vi "TestSSM.vi"(7 "TestBase.lvclass":refnum<class "TestBase.lvclass">, 10 "Script":string[](array[string])=["SamplerInitialize", "SamplerFetch,5000", "SyncSetTimedTrigger,Timed_1,0.1,0.1", "SamplerGetSamples", "Stop"], 11 "ModuleIDs":i32[](array[numeric])=[4140002, 4140002, 4140002, 4140002]) -> (0 "ErrorArray":errorcluster[](array[cluster]), 3 "Data":variant=variant(cluster{"dReadingArray":dbl[], "iActualPts":i32, "Timestamp":dbl}[] [{"dReadingArray"=array[9600 elements], "iActualPts"=9600, "Timestamp"=3606475867.981776}, {"dReadingArray"=array[9600 elements], "iActualPts"=9600, "Timestamp"=3606475867.981776}, {"dReadingArray"=array[9600 elements], "iActualPts"=9600, "Timestamp"=3606475867.981776}, {"dReadingArray"=array[9600 elements], "iActualPts"=9600, "Timestamp"=3606475867.981776}, {"dReadingArray"=array[9600 elements], "iActualPts"=9600, "Timestamp"=3606475867.981776}, {"dReadingArray"=array[9600 elements], "iActualPts"=9600, "Timestamp"=3606475867.981776}]))   [LabVIEW 2014, in "TestBase.lvclass"]
uses:
  TestBase.lvclass
  TestBase.lvclass/TestBase.ctl
  Accessors/Write ModuleIDs.vi
  Accessors/Write PluginPathArray.vi
  LV_Ini/Ini_lib.lvlib
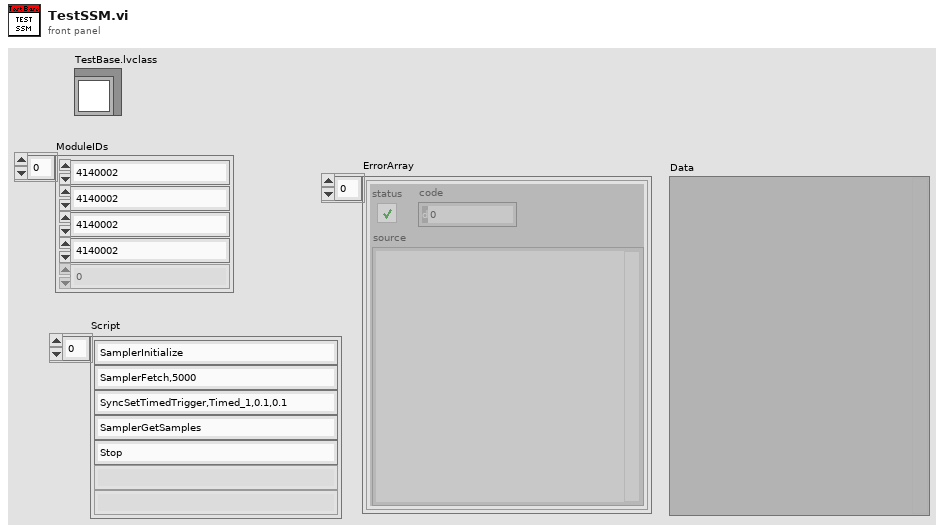
[diagram p1: front panel]
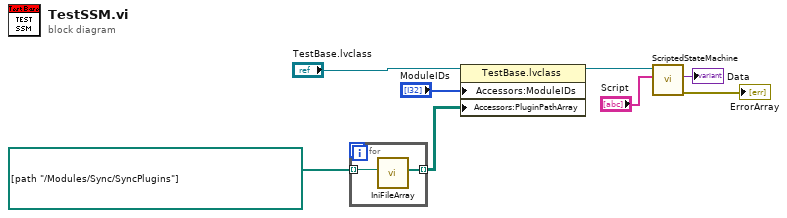
[diagram p0: block diagram]
diagram:
  n1 = for {
    tunnel: path[] [path "../Modules/Sync/SyncPlugins"] -> [w10] mode=indexing
    tunnel: [w9] -> w6 mode=indexing
    n2 = call "IniFileArray.vi"("Relative Path to Plugins"=w10) -> ("INIFilePaths"=w9:path[])  [unwired: 9 in, 1 out]
  }
  n3 = property class="TestBase.lvclass"(reference="TestBase.lvclass", "Accessors:ModuleIDs"="ModuleIDs", "Accessors:PluginPathArray"=w6) -> (reference out=w5:refnum<class "TestBase.lvclass">)  [unwired: 1 in, 1 out]
  n4 = call-dynamic "ScriptedStateMachine.vi"("Script"="Script", "TestBase.lvclass"=w5) -> ("ErrorArray"=→"ErrorArray":errorcluster[], "Data"=→"Data":variant)  [unwired: 7 in, 1 out]
